vi "hihb1.vi"(11 "file path 2":path=path "C:/luminartech/P11.2_Reflectance/src/Labview/bring_up/hihb1/hihb1_resp.txt") -> (3 "data array":dbl[](array[numeric]))   [LabVIEW 2018]
panel:
  out "opt_power":dbl
  out "LaserPower_min":dbl
  out "LaserPower_max":dbl
  out "LaserSeedTemp_min":dbl
  out "LaserSeedTemp_max":dbl
  out "size(s)":i32
  out "text 2":string[](array[string])
  out "line 2":string
  out "data table":dbl[][](array[numeric])
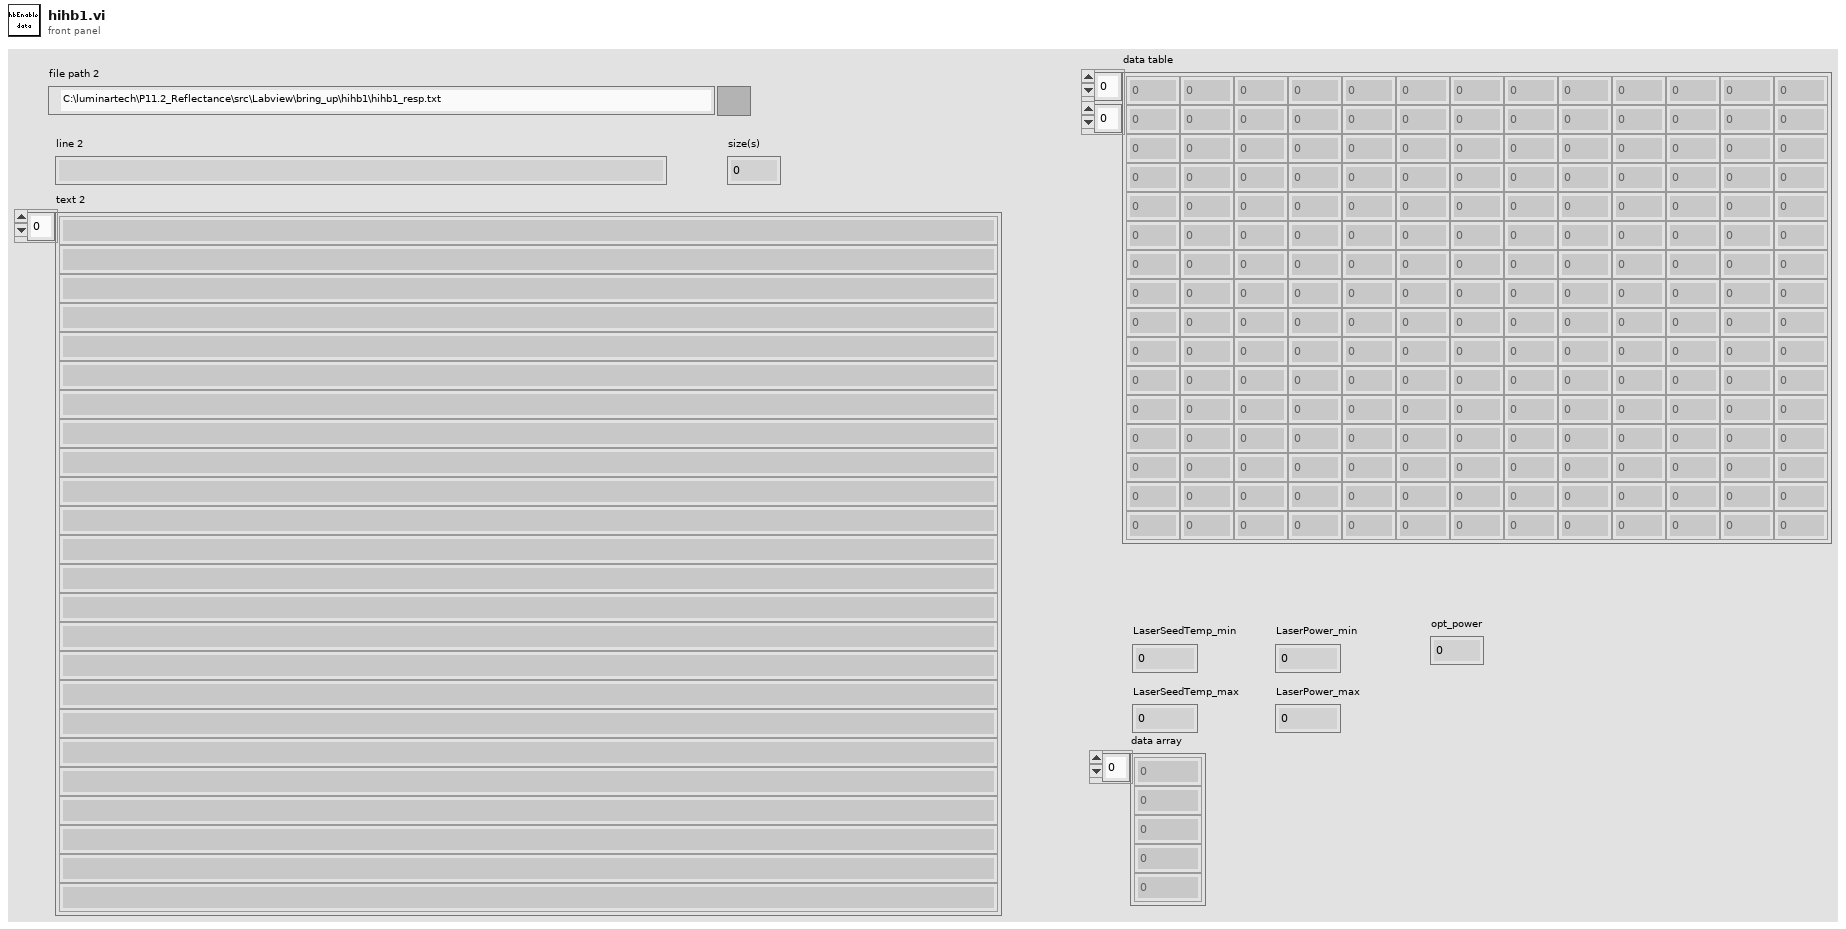
[diagram p1: front panel]
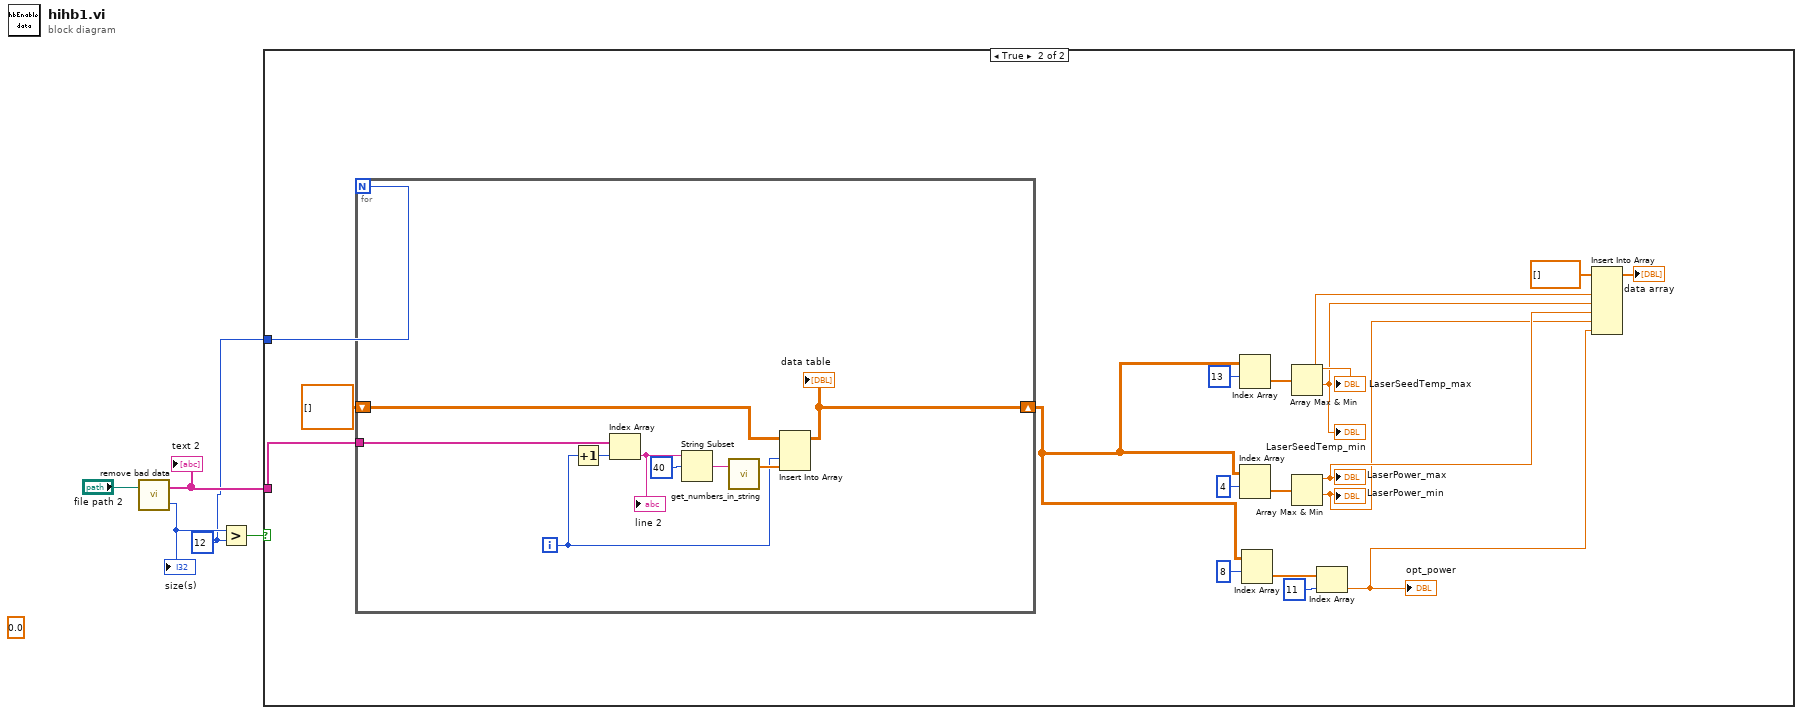
[diagram p0: block diagram]
diagram:
  (unwired) 0.0 ("COOL")
  w1 = 12 ("y")
  n1 = call "remove bad data.vi"("file path"="file path 2") -> ("size(s)"=w2:i32, "text 2"=w3:string[])  [unwired: 1 in]
  "text 2" <- w3
  "size(s)" <- w2
  n2 = Greater?(x=w2, y=w1) -> (0:w4:bool)
  n3 = case shown="True" w4 {
    tunnel: w3 -> [_ w22]
    tunnel: w1 -> [_ w21]
    frame False {
    }
    frame True {
      n4 = for {
        N: w21 -> [_]
        shift-right: [w28] -> w9
        shift-left: dbl[][] [] -> [w29]
        tunnel: w22 -> [w25]
        i -> [w26]
        n5 = Increment(x=w26) -> (x+1=w32:i32)
        n6 = Index Array(array=w25, index=w32) -> (element=w24:string)
        "line 2" <- w24
        n7 = String Subset(string=w24, offset (0)=40) -> (substring=w30:string)  [unwired: 1 in]
        n8 = call "get_numbers_in_string.vi"("String"=w30) -> ("Extracted Numbers"=w27:dbl[])  [unwired: 1 in, 1 out]
        n9 = Insert Into Array(array=w29, index (col)=w26, new element=w27) -> (w28:dbl[][])  [unwired: 1 in]
        "data table" <- w28
      }
      n10 = Index Array(array=w9, index (row)=13) -> (element=w20:dbl[])  [unwired: 1 in]
      n11 = Index Array(array=w9, index (row)=4) -> (element=w18:dbl[])  [unwired: 1 in]
      n12 = Index Array(array=w9, index (row)=8) -> (element=w8:dbl[])  [unwired: 1 in]
      n13 = Array Max & Min(array=w20) -> (max value=w16:dbl, min value=w15:dbl)  [unwired: 2 out]
      "LaserSeedTemp_max" <- w16
      "LaserSeedTemp_min" <- w15
      n14 = Array Max & Min(array=w18) -> (max value=w14:dbl, min value=w13:dbl)  [unwired: 2 out]
      "LaserPower_max" <- w14
      "LaserPower_min" <- w13
      n15 = Index Array(array=w8, index=11) -> (element=w6:dbl)
      "opt_power" <- w6
      n16 = Insert Into Array(array=dbl[] [], new element #1=w16, new element #2=w15, new element #3=w14, new element #4=w13, new element #5=w6) -> (→"data array":dbl[])  [unwired: 1 in]
    }
  }
